vi "Vending Machine SM.vi"() -> ()   [LabVIEW 2019]
panel:
  out "Row":i32
  in  "Menus":T1(array[cluster])
  out "Change":string="$0.00"
  out "Amount ($)":string="$0.00"
  out "error out":errorcluster={"status"=TRUE, "code"=7, "source"="Open/Create/Replace File in NI_LVConfig.lvlib:Load.vi->NI_LVConfig.lvlib:Open Config Data.vi->Configuration.vi->Vending Machine main.vi<APPEND>\nC:\\Users\\user\\Google 드라이브\\Jeonghwa\\Labview\\Labiview 2018\\Exam\\Configuration Data File.ini"}
  in  "error in":errorcluster
  out "Dispatch":bool
  in  "Return":bool
  in  "Deposit":bool
  in  "Selector":T2
  out "Elapsed time":dbl format="%#.2g"
  in  "Stop Button":bool
  # "Tip \n1. Insert the money \n2. Select the number\n3. Push the paid"
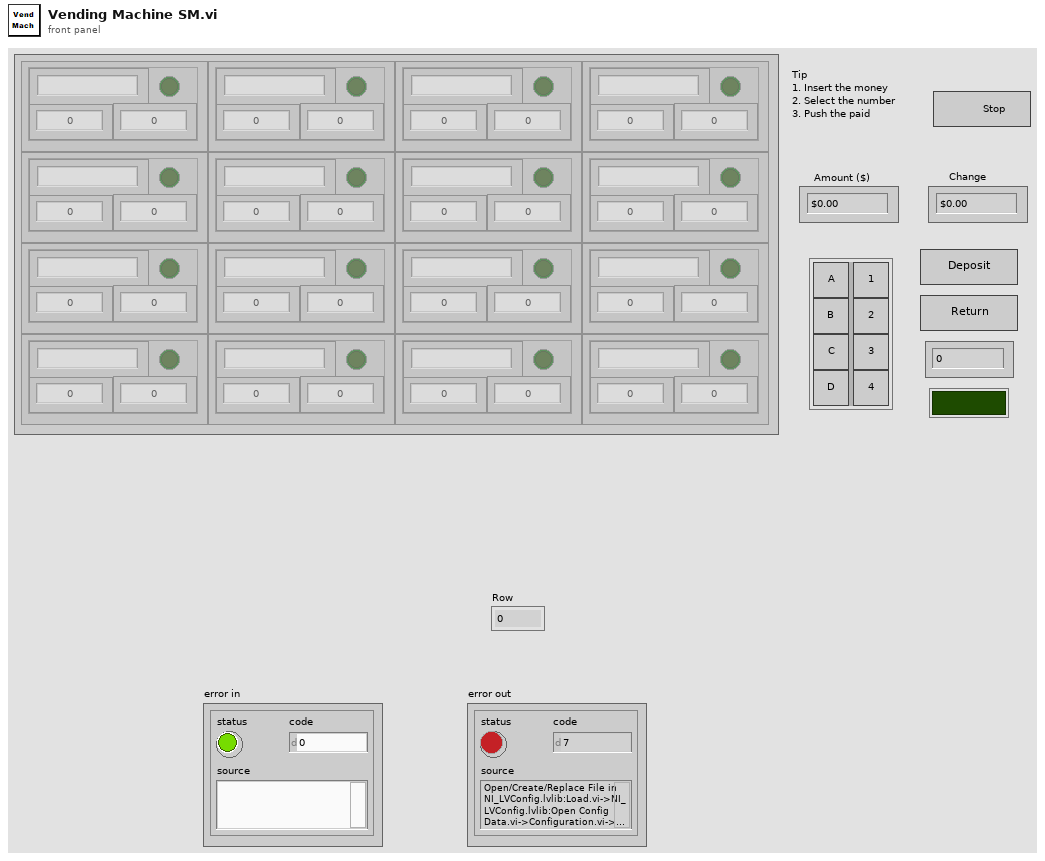
[diagram p1: front panel]
types:
  T1 = cluster{"Price":u32, "Name":string, "Left":u32, "Available":bool}[][]
  T2 = cluster{"A":bool, "B":bool, "C":bool, "D":bool, "1":bool, "2":bool, "3":bool, "4":bool}
  T3 = cluster{"Price":u32, "Name":string, "Left":u32, "Available":bool}
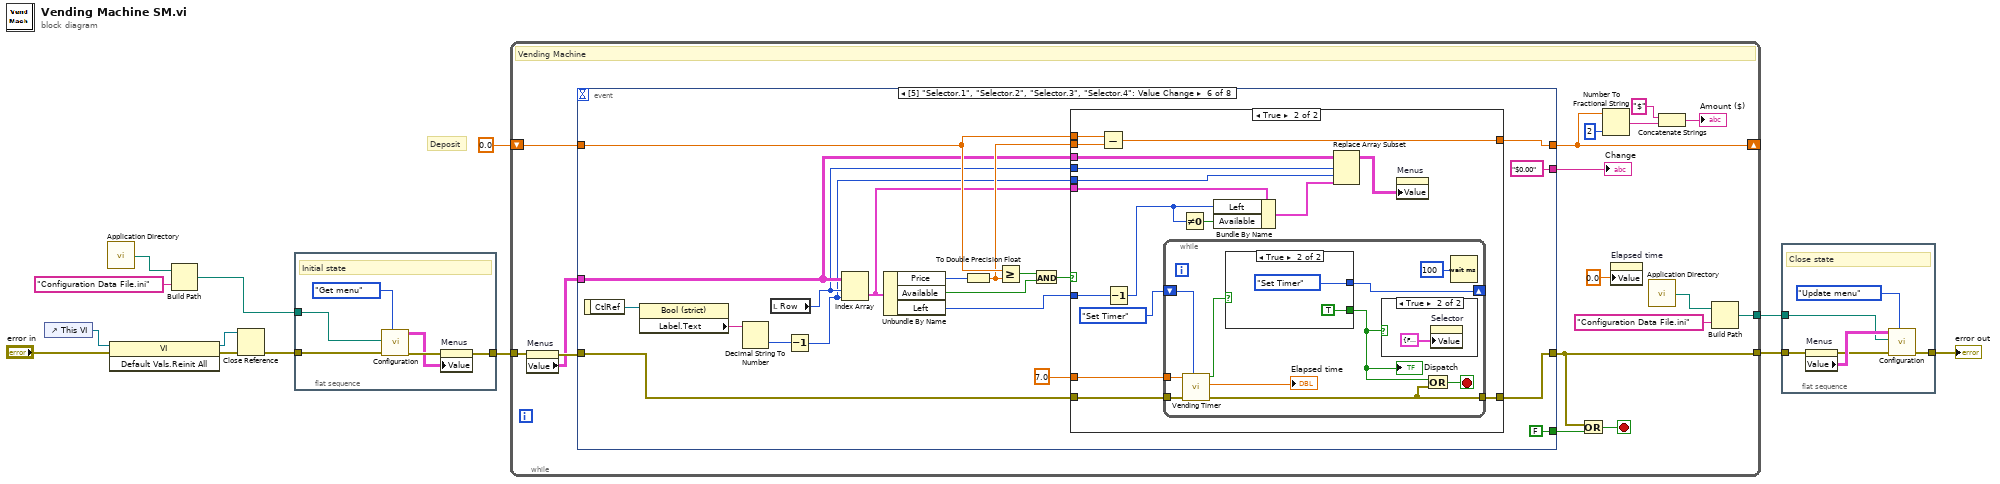
[diagram p0: block diagram]
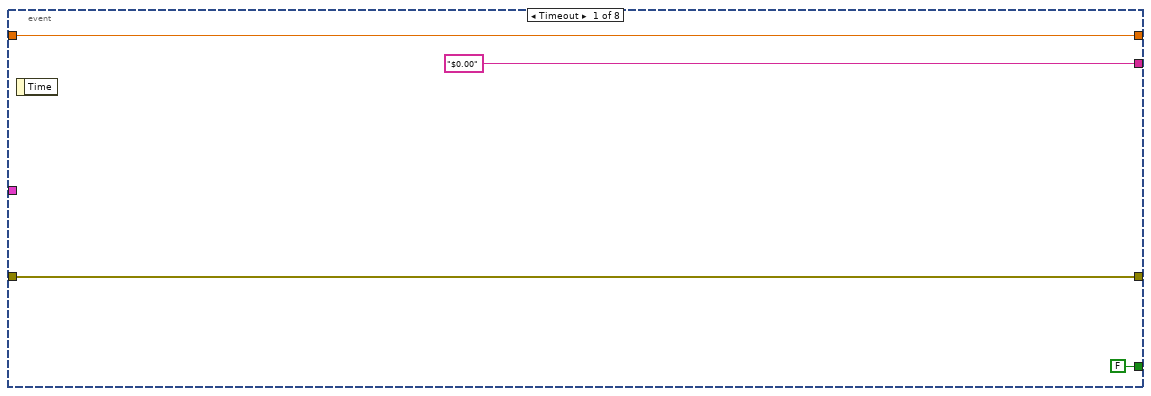
[diagram p2: hidden frame]
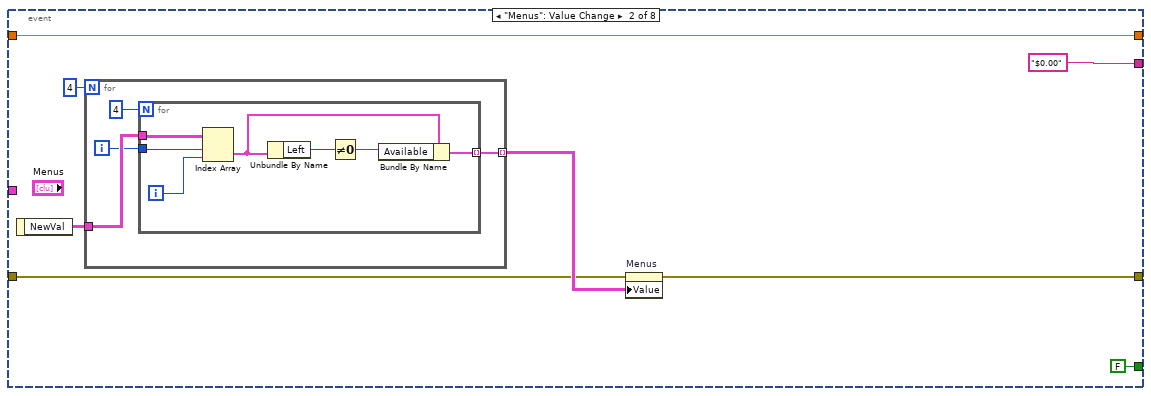
[diagram p3: hidden frame]
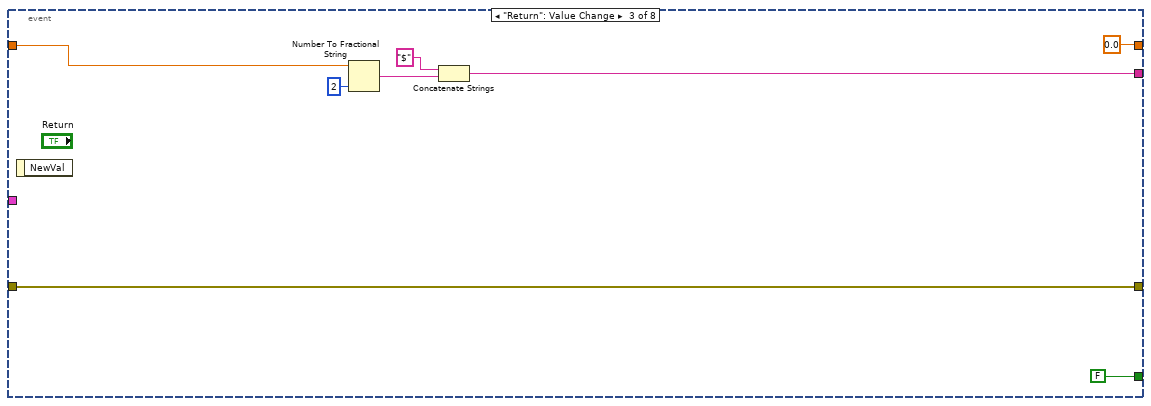
[diagram p4: hidden frame]
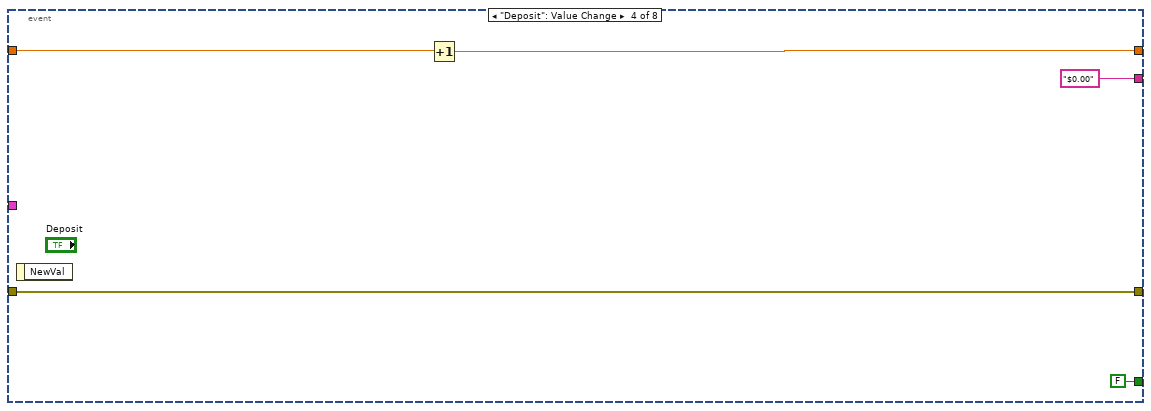
[diagram p5: hidden frame]
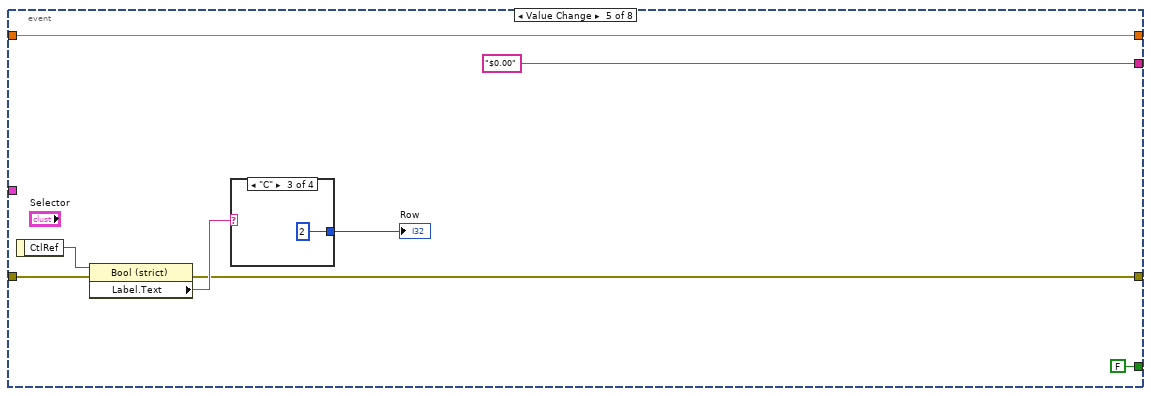
[diagram p6: hidden frame]
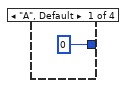
[diagram p7: hidden frame]
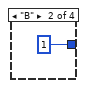
[diagram p8: hidden frame]
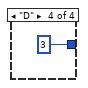
[diagram p9: hidden frame]
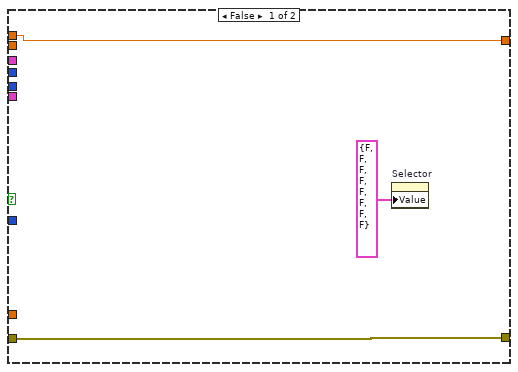
[diagram p10: hidden frame]
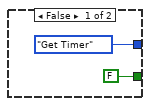
[diagram p12: hidden frame]
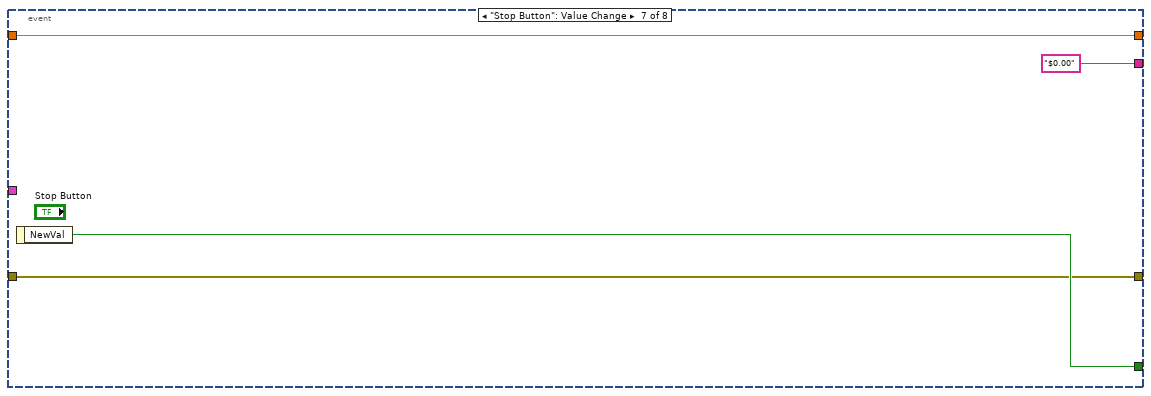
[diagram p13: hidden frame]
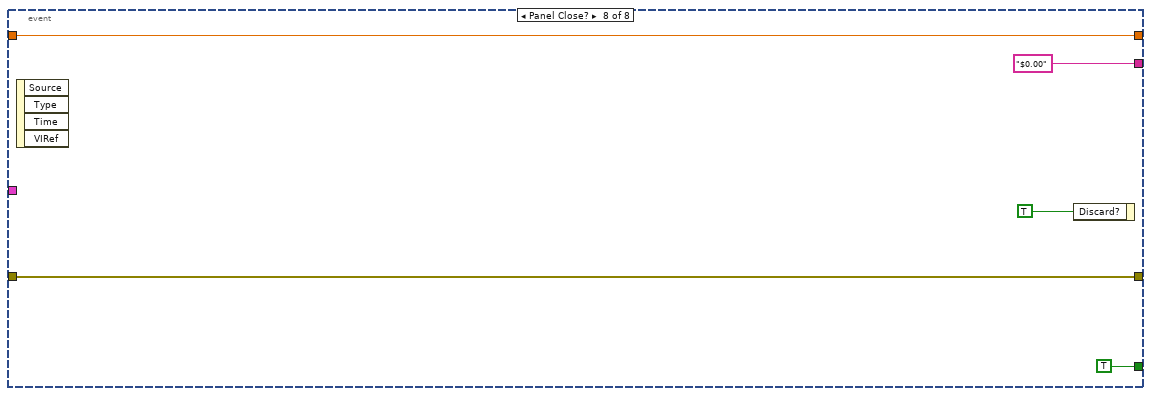
[diagram p14: hidden frame]
diagram:
  # "Deposit"
  n1 = control-ref of="This VI"() -> (w13:refnum<vi>)
  n2 = call <vilib>:"Application Directory.vi"() -> ("Application Directory"=w4:path)
  n3 = invoke class="VI" method="Default Vals.Reinit All"(reference=w13, error in="error in") -> (reference out=w12:refnum<vi>, error out=w11:errorcluster)  [unwired: 1 in, 1 out]
  n4 = Build Path(base path=w4, name or relative path="Configuration Data File.ini") -> (appended path=w2:path)
  n5 = Close Reference(reference=w12, error in (no error)=w11) -> (error out=w7:errorcluster)
  n6 = flat-sequence {
    tunnel: [w16] -> w8
    tunnel: w7 -> [w17]
    tunnel: w2 -> [w14]
    frame #0 {
      # "Initial state"
      n7 = call "Configuration.vi"("Get/Set"=enum16{"Get menu", "Update menu"}."Get menu" ("Get/Update"), "Error In"=w17, "Path"=w14) -> ("Error Out"=w18:errorcluster, "Menus out"=w15:T1)  [unwired: 7 in]
      n8 = property on="Menus" class="Arr (strict)"(error in=w18, "Value"=w15) -> (error out=w16:errorcluster)  [unwired: 1 in, 1 out]
    }
  }
  n9 = while {
    tunnel: w8 -> [w25]
    shift-right: [w28] -> _
    shift-left: 0.0 -> [w34]
    tunnel: [w27] -> w5
    tunnel: [w20] -> w1
    stop <- w36 stop-if-true
    # "Vending Machine"
    n10 = property on="Menus" class="Arr (strict)"(error in=w25) -> (error out=w24:errorcluster, "Value"=w23:T1)  [unwired: 1 in, 1 out]
    n11 = event shown="[5] \"Selector.1\", \"Selector.2\", \"Selector.3\", \"Selector.4\": Value Change" {
      selector: _ -> [_ _ _ _ _ _ _ _]
      dyn-events: _ -> [_ _ _ _ _ _ _ _]
      timeout: _ -> [_ _ _ _ _ _ _ _]
      tunnel: [FALSE ("NewVal") FALSE ("NewVal") FALSE ("NewVal") FALSE ("NewVal") FALSE ("NewVal") FALSE ("NewVal") w142 TRUE ("NewVal")] -> w33
      tunnel: ["$0.00" "$0.00" w61 "$0.00" "$0.00" "$0.00" "$0.00" "$0.00"] -> w35
      tunnel: w34 -> [w39 w45 w62 w71 w76 w94 w140 w144]
      tunnel: [w38 w42 w60 w69 w78 w91 w139 w143] -> w27
      tunnel: w23 -> [_ _ _ _ _ w89 _ _]
      tunnel: w24 -> [w38 w43 w60 w69 w77 w92 w139 w143]
      tunnel: [w39 w45 0.0 w70 w76 w86 w140 w144] -> w28
      event Timeout {
        n12 = event-data() -> ()  [unwired: 1 in, 1 out]
      }
      event "Menus": Value Change {
        n13 = event-data() -> ("NewVal"=w48:T1)  [unwired: 1 in]
        n14 = for {
          N: 4 -> [_]
          tunnel: w48 -> [w52]
          tunnel: [w50] -> w44 mode=indexing
          i -> [w51]
          n15 = for {
            N: 4 -> [_]
            tunnel: w52 -> [w58]
            tunnel: w51 -> [w59]
            tunnel: [w55] -> w50 mode=indexing
            i -> [w57]
            n16 = Index Array(array=w58, index (row)=w59, index (col)=w57) -> (element=w56:T3)
            n17 = Unbundle By Name(w56) -> ("Left"=w54:u32)
            n18 = Not Equal To 0?(x=w54) -> (x != 0?=w53:bool)
            n19 = Bundle By Name(cluster=w56, "Available"=w53) -> (w55:T3)
          }
        }
        n20 = property on="Menus" class="Arr (strict)"(error in=w43, "Value"=w44) -> (error out=w42:errorcluster)  [unwired: 1 in, 1 out]
      }
      event "Return": Value Change {
        n21 = event-data() -> ()  [unwired: 1 in, 1 out]
        n22 = Number To Fractional String(number=w62, precision (6)=i16 2) -> (F-format string=w63:string)  [unwired: 2 in]
        n23 = Concatenate Strings("$" ("string"), w63) -> (w61:string)
      }
      event "Deposit": Value Change {
        n24 = event-data() -> ()  [unwired: 1 in, 1 out]
        n25 = Increment(x=w71) -> (x+1=w70:dbl)
      }
      event "Selector.A", "Selector.B", "Selector.C", "Selector.D": Value Change {
        n26 = event-data() -> ("CtlRef"=w80:refnum<vi>)  [unwired: 1 in]
        n27 = property class="Bool (strict)"(reference=w80, error in=w77) -> (error out=w78:errorcluster, "Label.Text"=w79:string)  [unwired: 1 out]
        n28 = case shown="\"C\"" w79 {
          tunnel: [0 1 2 3] -> w74
          frame "A", Default {
          }
          frame "B" {
          }
          frame "C" {
          }
          frame "D" {
          }
        }
        "Row" <- w74
      }
      event "Selector.1", "Selector.2", "Selector.3", "Selector.4": Value Change {
        n29 = event-data() -> ("CtlRef"=w104:refnum<vi>)  [unwired: 1 in]
        n30 = property class="Bool (strict)"(reference=w104) -> ("Label.Text"=w103:string)  [unwired: 1 in, 2 out]
        n31 = Decimal String To Number(string=w103) -> (number=w102:i32)  [unwired: 2 in, 1 out]
        n32 = local read "Row"() -> (w88:i32)
        n33 = Decrement(x=w102) -> (x-1=w87:i32)
        n34 = Index Array(array=w89, index (row)=w88, index (col)=w87) -> (element=w90:T3)
        n35 = Unbundle By Name(w90) -> ("Price"=w99:u32, "Available"=w98:bool, "Left"=w95:u32)
        n36 = To Double Precision Float(number=w99) -> (double precision float=w93:dbl)
        n37 = Greater Or Equal?(x=w94, y=w93) -> (x >= y?=w100:bool)
        n38 = And(x=w100, y=w98) -> (x .and. y?=w96:bool)
        n39 = case shown="True" w96 {
          tunnel: [w107 w123] -> w91
          tunnel: 7.0 -> [_ w122]
          tunnel: w92 -> [w107 w120]
          tunnel: w94 -> [w105 w118]
          tunnel: w93 -> [_ w119]
          tunnel: w95 -> [_ w115]
          tunnel: w90 -> [_ w114]
          tunnel: w89 -> [_ w112]
          tunnel: w88 -> [_ w111]
          tunnel: w87 -> [_ w110]
          tunnel: [w105 w108] -> w86
          frame False {
            n40 = property on="Selector" class="Clust (strict)"("Value"=T2 {"A"=FALSE, "B"=FALSE, "C"=FALSE, "D"=FALSE, "1"=FALSE, "2"=FALSE, "3"=FALSE, "4"=FALSE} ("Selector")) -> ()  [unwired: 2 in, 2 out]
          }
          frame True {
            n41 = Subtract(x=w118, y=w119) -> (x-y=w108:dbl)
            n42 = Decrement(x=w115) -> (x-1=w116:u32)
            n43 = while {
              shift-right: [w131] -> _
              shift-left: enum16{"Get Timer", "Set Timer"}."Set Timer" ("Set/Get") -> [w129]
              tunnel: [w125] -> w123
              tunnel: w122 -> [w127]
              tunnel: w120 -> [w126]
              stop <- w128 stop-if-true
              n44 = call "Vending Timer.vi"("Set/Get"=w129, "Error In"=w126, "Target Time"=w127) -> ("Error Out"=w125:errorcluster, "Elapsed Time"=→"Elapsed time":dbl, "Elapsed?"=w133:bool)  [unwired: 4 in]
              n45 = case shown="True" w133 {
                tunnel: [enum16{"Get Timer", "Set Timer"}."Get Timer" ("Set/Get") enum16{"Get Timer", "Set Timer"}."Set Timer" ("Set/Get")] -> w131
                tunnel: [FALSE ("Dispatch") TRUE ("Dispatch")] -> w124
                frame False {
                }
                frame True {
                }
              }
              "Dispatch" <- w124
              n46 = case shown="True" w124 {
                frame False {
                }
                frame True {
                  n47 = property on="Selector" class="Clust (strict)"("Value"=T2 {"A"=FALSE, "B"=FALSE, "C"=FALSE, "D"=FALSE, "1"=FALSE, "2"=FALSE, "3"=FALSE, "4"=FALSE} ("Selector")) -> ()  [unwired: 2 in, 2 out]
                }
              }
              n48 = Or(x=w124, y=w125) -> (x .or. y?=w128:bool)
              n49 = Wait (ms)(milliseconds to wait=u32 100) -> ()  [unwired: 1 out]
            }
            n50 = Not Equal To 0?(x=w116) -> (x != 0?=w117:bool)
            n51 = Bundle By Name(cluster=w114, "Left"=w116, "Available"=w117) -> (w113:T3)
            n52 = Replace Array Subset(array=w112, new element=w113, index (row)=w111, index (col)=w110) -> (w109:T1)
            n53 = property on="Menus" class="Arr (strict)"("Value"=w109) -> ()  [unwired: 2 in, 2 out]
          }
        }
      }
      event "Stop Button": Value Change {
        n54 = event-data() -> ("NewVal"=w142:bool)  [unwired: 1 in]
      }
      event Panel Close? {
        n55 = event-data() -> ()  [unwired: 1 in, 4 out]
        n56 = event-data("Discard?"=TRUE) -> ()  [unwired: 1 in, 1 out]
      }
    }
    "Change" <- w35
    n57 = Or(x=w27, y=w33) -> (x .or. y?=w36:bool)
    n58 = Number To Fractional String(number=w28, precision (6)=i16 2) -> (F-format string=w32:string)  [unwired: 2 in]
    n59 = property on="Elapsed time" class="DigNum (strict)"("Value"=0.0 ("Elapsed time")) -> ()  [unwired: 2 in, 2 out]
    n60 = call <vilib>:"Application Directory.vi"() -> ("Application Directory"=w22:path)
    n61 = Concatenate Strings("$" ("string"), w32) -> (→"Amount ($)":string)
    n62 = Build Path(base path=w22, name or relative path="Configuration Data File.ini") -> (appended path=w20:path)
  }
  n63 = flat-sequence {
    tunnel: [w152] -> w10
    tunnel: w5 -> [w149]
    tunnel: w1 -> [w148]
    frame #0 {
      # "Close state"
      n64 = property on="Menus" class="Arr (strict)"(error in=w149) -> (error out=w150:errorcluster, "Value"=w151:T1)  [unwired: 1 in, 1 out]
      n65 = call "Configuration.vi"("Get/Set"=enum16{"Get menu", "Update menu"}."Update menu" ("Get/Update"), "Error In"=w150, "Path"=w148, "Menus"=w151) -> ("Error Out"=w152:errorcluster)  [unwired: 6 in, 1 out]
    }
  }
  "error out" <- w10
